vi "Subscribe.vi"(5 "Message Transport Interface":refnum<class "Message Transport Interface.lvclass">, 6 "Subscriber Name":string, 7 "Topic Name":string, 8 "error in (no error)":errorcluster, 11 "Message Broker in":refnum<class "Message Broker.lvclass">) -> (0 "error out":errorcluster, 2 "Topic Actor Created?":bool, 3 "Message Broker out":refnum<class "Message Broker.lvclass">)   [LabVIEW 2016, in "Stream Mediator.lvlib" / "Message Broker.lvclass"]
doc: "--\nCopyright © 2017 Composed SystemsI All rights reserved.\n\nAuthor: Jon McBee <jon.mcbee@composed.io>\n\nThis library is provided \"AS IS\" ,WITHOUT WARRANTIES OR\nCONDITIONS OF ANY KIND, either express or implied.\n\nComposed Systems -- composed.io\n\nStream 0.0.1.1\nJon McBee - Composed Systems\nCopyright (c) 2017, Composed Systems"
uses:
  <userlib>/Composed Systems/Stream/Mediator/Classes/Message Broker/Message Broker.lvclass
  <userlib>/Composed Systems/Stream/Mediator/Classes/Message Transport Interface/Message Transport Interface.lvclass
  <userlib>/Composed Systems/Stream/Mediator/Classes/Topic Actor Subscribe Command/Topic Actor Subscribe Command.lvclass
  C:/Program Files (x86)/National Instruments/LabVIEW 2016/user.lib/Composed Systems/Stream/Mediator/Classes/Message Interface/Message Interface.lvclass
  <userlib>/Composed Systems/Stream/Mediator/Classes/Message Broker/Message Broker.lvclass/Message Broker.ctl
  <userlib>/Composed Systems/Stream/Mediator/Classes/Message Transport Queue/Message Transport Queue.lvclass
  <userlib>/Composed Systems/Stream/Mediator/Classes/Topic Actor Look Up Table/Topic Actor Look Up Table.lvclass
  <userlib>/Composed Systems/Stream/Mediator/Classes/Topic Actor Descriptor/Topic Actor Descriptor.lvclass
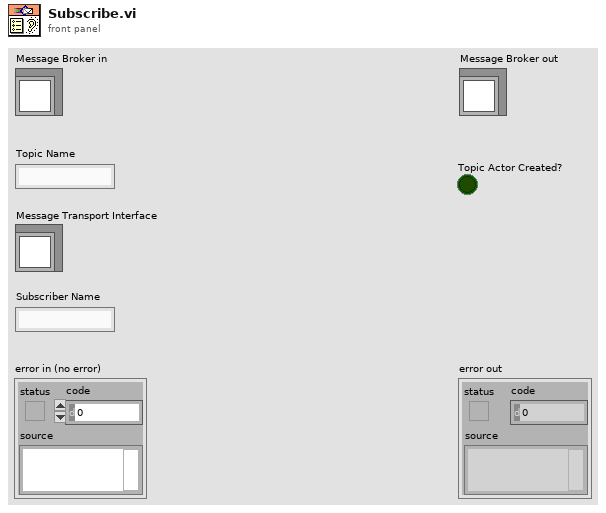
[diagram p1: front panel]
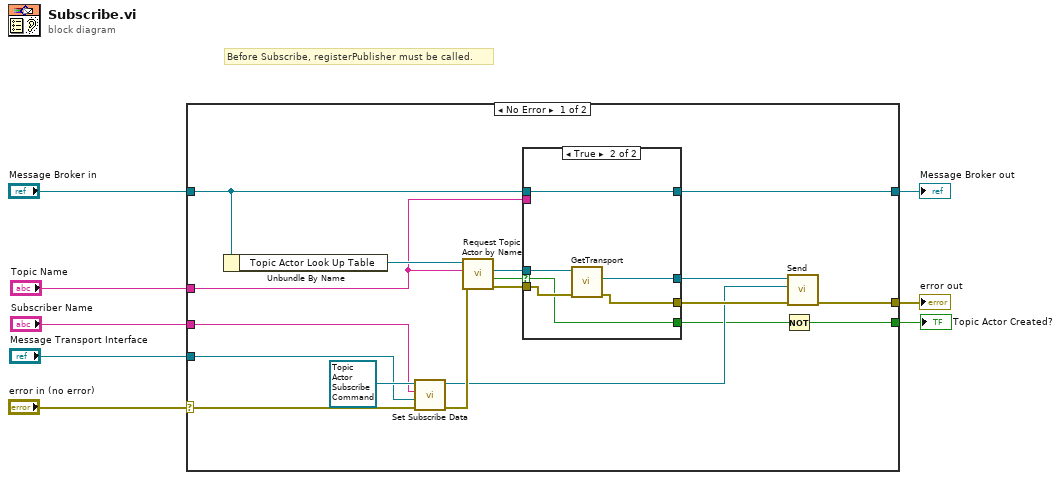
[diagram p0: block diagram]
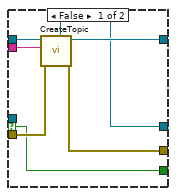
[diagram p2: hidden frame]
diagram:
  # "Before Subscribe, registerPublisher must be called."
  n1 = case shown="No Error" "error in (no error)" {
    selector: "error in (no error)" -> [w19 w41]
    tunnel: [w15 w41] -> w7
    tunnel: [w23 w40] -> w5
    tunnel: "Message Broker in" -> [w24 w40]
    tunnel: "Topic Name" -> [w17 _]
    tunnel: "Message Transport Interface" -> [w16 _]
    tunnel: "Subscriber Name" -> [w11 _]
    tunnel: [w9 _] -> w1
    frame No Error {
      n2 = Unbundle By Name(w24) -> ("Topic Actor Look Up Table"=w26:refnum<class "Topic Actor Look Up Table.lvclass">)
      n3 = call <userlib>:"Set Subscribe Data.vi"("error in (no error)"=w19, "Message Transport Interface"=w16, "Subscriber Name"=w11, "Topic Actor Subscribe Command in"=refnum<class "Topic Actor Subscribe Command.lvclass"> refnum ("Topic Actor Subscribe Command.lvclass")) -> ("error out"=w18:errorcluster, "Topic Actor Subscribe Command out"=w12:refnum<class "Topic Actor Subscribe Command.lvclass">)  [unwired: 6 in]
      n4 = call <userlib>:"Request Topic Actor by Name.vi"("error in (no error)"=w18, "Topic Actor"=w17, "Topic Actor Look Up Table in"=w26) -> ("error out"=w21:errorcluster, "Found?"=w25:bool, "Topic Actor Descriptor"=w22:refnum<class "Topic Actor Descriptor.lvclass">)  [unwired: 5 in, 1 out]
      n5 = case shown="True" w25 {
        selector: w25 -> [w27 w34]
        tunnel: [w32 w39] -> w23
        tunnel: w24 -> [w33 w39]
        tunnel: [w29 w37] -> w14
        tunnel: w22 -> [_ w36]
        tunnel: w17 -> [w31 _]
        tunnel: w21 -> [w30 w38]
        tunnel: [w28 w35] -> w13
        tunnel: [w27 w34] -> w10
        frame False {
          n6 = call-dynamic "CreateTopic.vi"("error in (no error)"=w30, "Topic Name"=w31, "Message Broker in"=w33) -> ("error out"=w29:errorcluster, "Message Broker out"=w32:refnum<class "Message Broker.lvclass">, "Transport"=w28:refnum<class "Message Transport Queue.lvclass">)  [unwired: 5 in, 1 out]
        }
        frame True {
          n7 = call <userlib>:"GetTransport.vi"("error in (no error)"=w38, "Topic Actor Descriptor in"=w36) -> ("error out"=w37:errorcluster, "Transport"=w35:refnum<class "Message Transport Queue.lvclass">)  [unwired: 7 in, 1 out]
        }
      }
      n8 = Not(x=w10) -> (.not. x?=w9:bool)
      n9 = call-dynamic "Send.vi"("error in (no error)"=w14, "Message"=w12, "Message Transport Queue in"=w13) -> ("error out"=w15:errorcluster)  [unwired: 6 in, 2 out]
    }
    frame Error {
    }
  }
  "error out" <- w7
  "Message Broker out" <- w5
  "Topic Actor Created?" <- w1
